vi "Construct.vi"(8 "error in (no error)":errorcluster, 9 "Topic":string, 10 "Subscription ID":u64, 11 "SubscriptionDetailsParent in":refnum<class "SubscriptionDetailsParent.lvclass">) -> (0 "error out":errorcluster, 3 "SubscriptionDetailsParent out":refnum<class "SubscriptionDetailsParent.lvclass">)   [LabVIEW 2020, in "wamplv.lvlib" / "SubscriptionDetailsParent.lvclass"]
uses:
  SubscriptionDetailsParent.lvclass
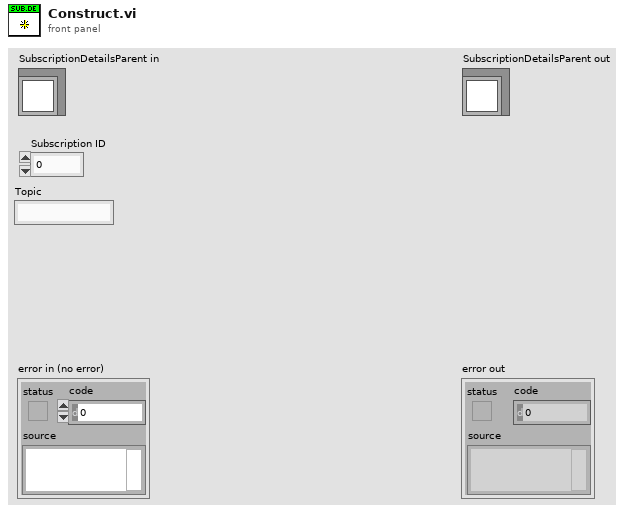
[diagram p1: front panel]
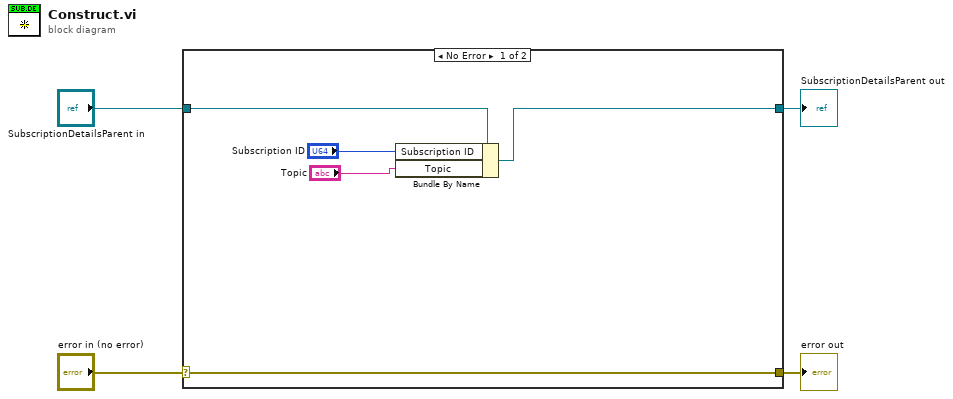
[diagram p0: block diagram]
diagram:
  n1 = case shown="No Error" "error in (no error)" {
    selector: "error in (no error)" -> [w9 w11]
    tunnel: [w9 w11] -> w3
    tunnel: [w7 w10] -> w1
    tunnel: "SubscriptionDetailsParent in" -> [w8 w10]
    frame No Error {
      n2 = Bundle By Name(cluster=w8, "Subscription ID"="Subscription ID", "Topic"="Topic") -> (w7:refnum<class "SubscriptionDetailsParent.lvclass">)
    }
    frame Error {
    }
  }
  "error out" <- w3
  "SubscriptionDetailsParent out" <- w1
